vi "service.vi"(8 "error in (no error)":errorcluster, 11 "system.logging in":refnum<class "system.logging.lvclass">) -> (0 "error out":errorcluster)   [LabVIEW 2021, in "system.logging.lvclass"]
uses:
  system.logging.lvclass
  system.logging.lvclass/system.logging.ctl
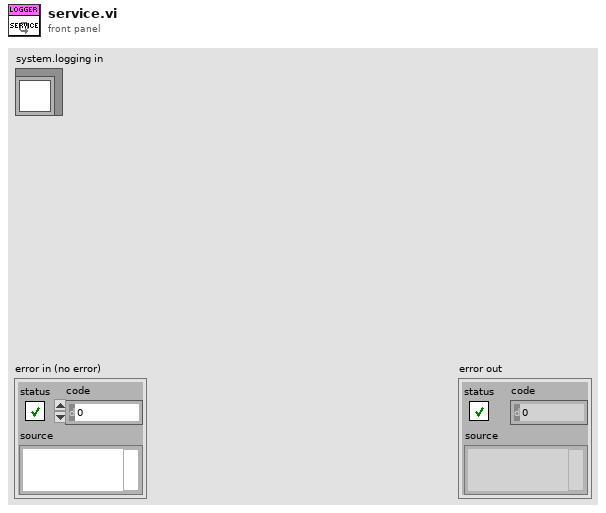
[diagram p1: front panel]
types:
  T1 = typedef "system.logging.lvclass/log_entry.ctl" = cluster{"severity":T2, "message":string, "origin":string, "datetime":timestamp}
  T2 = typedef "system.logging.lvclass/severity.ctl" = enum8{"trace", "debug", "info", "warning", "error"}
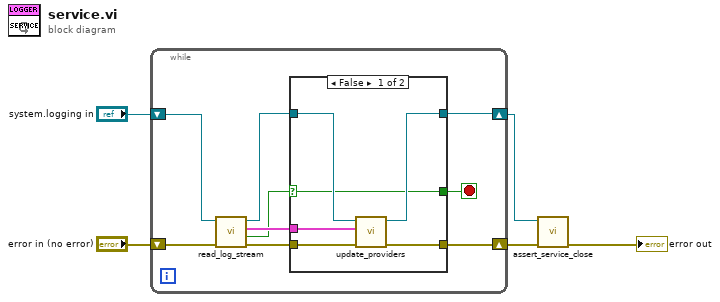
[diagram p0: block diagram]
diagram:
  n1 = while {
    shift-right: [w14] -> w3
    shift-left: "error in (no error)" -> [w9]
    shift-right: [w13] -> w2
    shift-left: "system.logging in" -> [w10]
    stop <- w6 stop-if-true
    n2 = call "read_log_stream.vi"("error in (no error)"=w9, "system.logging in"=w10) -> ("error out"=w11:errorcluster, "abort?"=w7:bool, "log_entry"=w8:T1, "system.logging out"=w12:refnum<class "system.logging.lvclass">)  [unwired: 6 in]
    n3 = case shown="False" w7 {
      selector: w7 -> [w15 w22]
      tunnel: [w20 w21] -> w14
      tunnel: [w19 w23] -> w13
      tunnel: w12 -> [w18 w23]
      tunnel: w11 -> [w17 w21]
      tunnel: w8 -> [w16 _]
      tunnel: [w15 w22] -> w6
      frame False {
        n4 = call "update_providers.vi"("error in (no error)"=w17, "log_entry"=w16, "system.logging in"=w18) -> ("error out"=w20:errorcluster, "system.logging out"=w19:refnum<class "system.logging.lvclass">)  [unwired: 7 in]
      }
      frame True {
      }
    }
  }
  n5 = call "assert_service_close.vi"("error in (no error)"=w3, "system.logging in"=w2) -> ("error out"=→"error out":errorcluster)  [unwired: 9 in]
